vi "testWrongCount.vi"() -> ()   [LabVIEW 2019, in "AssertionTest.lvlib" / "AssertNotCount.lvlib"]
uses:
  AssertNotCount.lvlib
  Assertion/Assertion.lvlib
panel:
  out "error out":errorcluster
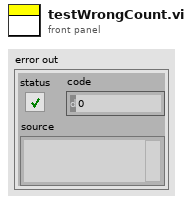
[diagram p1: front panel]
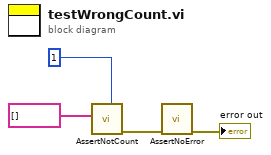
[diagram p0: block diagram]
diagram:
  n1 = call "AssertNotCount.vi"("Expected"=1, "Haystack"=string[] []) -> ("error out"=w1:errorcluster)  [unwired: 9 in]
  n2 = call "AssertNoError.vi"("error in (no error)"=w1) -> ("error out"=→"error out":errorcluster)  [unwired: 10 in]
